vi "Dashboard Main.vi"() -> ()   [LabVIEW 2015]
uses:
  <vilib>/Utility/miscctls.llb/LVRowAndColumnTypeDef.ctl
  <vilib>/event_ctls.llb/eventvkey.ctl
  <vilib>/Rock Robotics/WPI/Dashboard/WPI_DashboardLogging Global.vi
  <vilib>/Rock Robotics/Network Tables/NT Read Numeric Array.vi
  <vilib>/Rock Robotics/Network Tables/NT Read Boolean Array.vi
  <vilib>/Rock Robotics/Network Tables/NT Read Boolean.vi
  <vilib>/Utility/config.llb/Write Key (String).vi
  <vilib>/Utility/config.llb/Write Key (I32).vi
  <vilib>/Utility/config.llb/NI_LVConfig.lvlib
panel:
  in  "TCP":refnum<k5>
  in  "Rec Mode":enum32{"Stop", "Record", "Playback"}(radio)
  in  "Vision":u16(ring)=2 items=["Camera Off", "USB Camera SW", "USB Camera HW", "IP Camera"]
  out "Camera IP":string
  out "Image Message":string="Timeout in Camera Communications"
  in  "Dashboard Tab":T1(tab)
  out "Selected Auto Scheme":string
  out "Gyro":dbl(knob) scale=0.0..360.0
  out "xpos":dbl(slide) scale=-1.0..1.0
  out "target3":bool
  out "target2":bool
  out "target1":bool
  out "NT Connection":bool
  in  "Camera Settings":T2={"Frame Rate"=30, "Compression"=30, "Size"=1} {"Frame Rate" scale=1.0..30.0; "Size" items=["640x480", "320x240", "160x120"]}
  out "MotorChart R":cluster{"Numeric":dbl, "Numeric":dbl}(graph)
  out "MotorChart L":T3(graph)
  out "MotorSliders R":cluster{"MotorSlide1":dbl, "MotorSlide2":dbl} {"MotorSlide2" scale=-1.0..1.0 scale format="%#_2e"; "MotorSlide1" scale=-1.0..1.0 scale format="%#_2e"}
  out "MotorSliders L":T4 {"MotorSlide4 2" scale=0.0..14.0 scale format="%#_2e"; "MotorSlide2" scale=-1.0..1.0 scale format="%#_2e"; "MotorSlide1" scale=-1.0..1.0 scale format="%#_2e"}
  out "JS1 Z":dbl(slide) scale=-1.0..1.0 scale format="%#_2e"
  out "JS1 Graph":cluster{"X":dbl, "Y":dbl}[](graph)
  out "JS1 Buttons":T5
  out "JS2 Z":dbl(slide) scale=-1.0..1.0 scale format="%#_2e"
  out "JS2 Graph":cluster{"X":dbl, "Y":dbl}[](graph)
  out "JS2 Buttons":T5
  out "Mode":T6(ring)=enum."Auto Disabled"
  in  "DB Camera Config":bool
  out "fps":dbl format="%#.1g"
  out "Mbps":dbl format="%#.1g"
  out "Mbps LED":bool
  out "Joystick":bool
  out "Ball":bool
  out "ArmLimit":bool
  out "Intake":bool
  out "Defense":bool
  out "Ldistance":dbl caption="Left"
  out "Rdistance":dbl caption="Right"
  in  "DB/String 9":string
  in  "DB/String 8":string
  in  "DB/String 7":string
  in  "DB/String 6":string
  in  "DB/String 5":string
  in  "DB/String 4":string
  in  "DB/String 3":string
  in  "DB/String 2":string
  in  "DB/String 1":string
  in  "DB/String 0":string
  in  "DB/Slider 0":dbl(slide) scale=0.0..5.0
  in  "DB/Slider 1":dbl(slide) scale=0.0..5.0
  in  "DB/Slider 2":dbl(slide) scale=0.0..5.0
  in  "DB/Slider 3":dbl(slide) scale=0.0..5.0
  out "DB/LED 3":bool
  out "DB/LED 2":bool
  out "DB/LED 1":bool
  out "DB/LED 0":bool
  in  "DB/Button 3":bool
  in  "DB/Button 2":bool
  in  "DB/Button 1":bool
  in  "DB/Button 0":bool caption="New Name"
  in  "BasicAutoParam":dbl[](array[numeric])=[46.0, 95.0, 195.0, 0.5] caption="Auto Params (low bar + others)"
  in  "SelEncoder":bool caption="Use which encoder?"
  in  "Kp":dbl=-0.5 caption="Run straight gain (Kp)"
  in  "Select Auto":string(combo) caption="Select Auto Options"
  in  "idealposition":dbl[](array[numeric])=[8.9, 0.1, 0.08, 0.05] caption="Ideal Position"
  in  "idealspeed":dbl[](array[numeric])=[0.55, 0.55] caption="Ideal Speed"
  out "target":dbl[](array[numeric]) caption="Target"
  in  "Test Slider":dbl(slide) scale=0.0..100.0 scale format="%#_3g"
  in  "On/Off":bool caption="Solenoid"
  in  "Test Name":u16(ring) items=["Select the test to run..."]
  in  "Test Tree":string(tree)
  in  "Motor":cluster{"Value":dbl, "Enable":bool} {"Value" scale=-1.0..1.0 scale format="%#_3g"}
  out "Progress":T7 {"Test Progress" scale=0.0..100.0}
  in  "Rev/Fwd":cluster{"Forward":bool, "Reverse":bool}
  in  "Test Ring":u16(ring) items=["Monochrome", "Color"]
  out "Cmd Status":string
  in  "Execute Command":bool
  in  "Command Params":string[][](table)
  in  "Command Selection":i32(listbox)
  in  "CheckList":i32(listbox)
  out "Tree":string(tree)
  out "Camera Image":T8(plugin-control)
  out "Background":bool
  # "Left"
  # "Front"
  # "Right"
  # "Battery"
  # "Approach distance (auto to defense)"
  # "Breach distance (across defense)"
  # "Travel distance (100\" beyond defense)"
  # "Clockwise turn time (seconds)\nLow bar = 0.5\nRough Terrian / Rock wall = 2.0\nMoat = 3.0"
  # "distance to target"
  # "# targets"
  # "distance to target"
  # "x deadband (close)"
  # "center x"
  # "x center"
  # "center y"
  # "x deadband (far)"
  # "drive speed"
  # "turn speed"
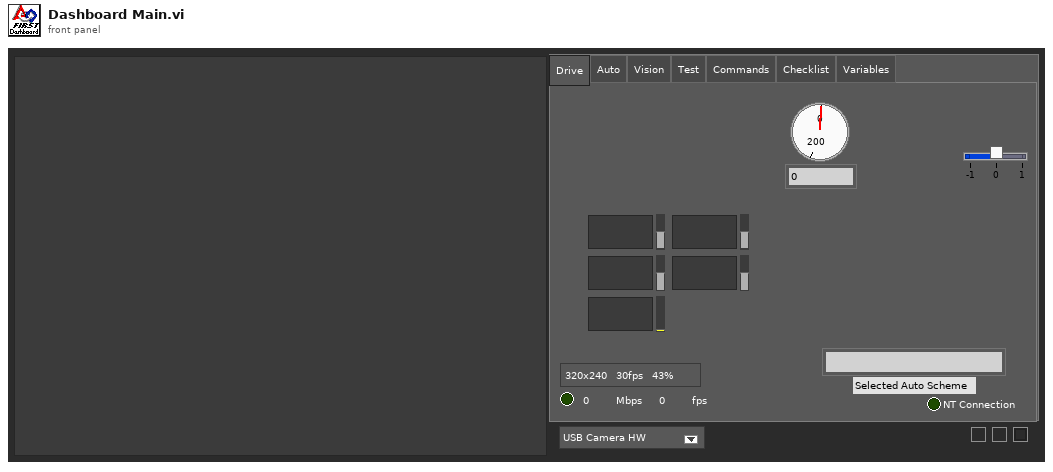
[diagram p1: front panel]
types:
  T1 = enum32{"Drive", "Basic", "Auto", "Vision", "Test", "Commands", "Checklist", "Variables"}
  T2 = cluster{"Frame Rate":i32, "Compression":i32, "Size":u16}
  T3 = cluster{"Numeric":dbl, "Numeric":dbl, "Battery V":dbl}
  T4 = cluster{"MotorSlide1":dbl, "MotorSlide2":dbl, "MotorSlide4 2":dbl}
  T5 = cluster{bool, bool, bool, bool, bool, bool, bool, bool, bool, bool, bool, bool}
  T6 = enum8{"Tele-Op Disabled", "Tele-Op Enabled", "Auto Disabled", "Auto Enabled", "Test Disabled", "Test Enabled", "Disconnected", "No Code", "E-Stop"}
  T7 = cluster{"Test Progress":u8, "Test Progress Text":string}
  T8 = typedef "IMAQ Image.ctl" = refnum<image>
  T9 = cluster{"IDs":cluster{"RPC field ID":u16, "Unique ID":u16}, "String":string}
  T10 = typedef "Image Type" = u32
  T11 = cluster{"Camera Image":refnum<vi>, "Dashboard Tab":refnum<vi>, "Background":refnum<vi>, "Vision":refnum<vi>, "Rec Mode":refnum<vi>, "Test Slider":refnum<vi>, "On/Off ":refnum<vi>, "Test Ring":refnum<vi>, "Rev/Fwd":refnum<vi>, "Test Name":refnum<vi>, "Motor":refnum<vi>, "Progress":refnum<vi>, "CheckList":refnum<vi>, "Tree":refnum<vi>, "Test Tree":refnum<vi>, "Command Params":refnum<vi>, "Command Selection":refnum<vi>, "Execute Command":refnum<vi>, "Cmd Status":refnum<vi>}
  T12 = cluster{"Error Strings":string, "Disable Counts":cluster{u16, u16}, "Rail Faults":cluster{u16, u16, u16}, "Robot IP":string, "DB Mode":u8, "Event Info":cluster{"Name":string, "Type":u8, "Number":u16, "Replay":u8}, "Camera Addr":string}
  T13 = cluster{"Storage":cluster{"Disk Free":u64, "RAM Block":u32, "RAM free":u32}, "CPU Utilization":cluster{"CPU % ISR":sgl, "CPU % Time Crit":sgl, "CPU % Timed Str":sgl, "CPU % High":sgl, "CPU % Above":sgl, "CPU % Normal":sgl, "CPU % Low":sgl}, "CAN":cluster{"% Bus Utilization":sgl, "Bus Off Cnt":u32, "TX_FIFO Full Cnt":u32, "Receive Error Cnt":u8, "Transmit Error Cnt":u8}, "HID":cluster{"HID Outputs":u32, "Rumble Low":u16, "Rumble High":u16}[]}
  T14 = cluster{"Status bits":cluster{"Test Mode":bool, "Autonomous":bool, "Enabled":bool, "Code Start":bool, "Brownout":bool, "Reserved 2":bool, "Reserved 3":bool, "E-Stop":bool}, "Code Trace":cluster{"Disabled":bool, "TeleOp":bool, "Auto":bool, "Test":bool}, "Controller Type":enum16{"unknown", "cRIO", "roboRio"}, "Code?":enum16{"unknown", "noCode", "code"}, "Battery V":dbl}
  T15 = cluster{"Control Bits":cluster{"TestMode":bool, "Autonomous":bool, "Enabled":bool, "FMS Present":bool, bool, bool, bool, "E-Stop":bool}, "Team Station ":u8, "Countdown":sgl, "Joystick Values":cluster{"Axes":dbl[], "Buttons":bool[], "POVs":i16[]}[]}
  T16 = cluster{"Axes":dbl[], "Buttons":bool[], "POVs":i16[]}[]
  T17 = cluster{"Axes":dbl[], "Buttons":bool[], "POVs":i16[]}
  T18 = cluster{"Buttons[0]":bool, "Buttons[1]":bool, "Buttons[2]":bool, "Buttons[3]":bool, "Buttons[4]":bool, "Buttons[5]":bool, "Buttons[6]":bool, "Buttons[7]":bool, "Buttons[8]":bool, "Buttons[9]":bool, "Buttons[10]":bool, "Buttons[11]":bool}
  T19 = typedef "NI_LVConfig.lvlib/Config Data RefNum.ctl" = refnum<k1>
  T20 = cluster{"Operation":enum16{"Update", "Clear"}, "Color Box":u32}[]
  T21 = typedef "eventvkey.ctl" = enum16{"ASCII", "Enter", "Return", "Shift", "Ctrl", "Alt", "Cmd", "Opt", "Caps", "NumLock", "Clear", "Break", "Up", "Down", "Left", "Right", "Insert", "Delete", "Home", "End", "PageUp", "PageDown", "Escape", "Help", "Pause", "ScrollLock", "F1", "F2", "F3", "F4", "F5", "F6", "F7", "F8", "F9", "F10", "F11", "F12", "F13", "F14", "F15", "F16", "F17", "F18", "F19", "F20", "F21", "F22", "F23", "F24", "Play", "VolumeUp", "VolumeDown", "Mute", "Two Byte Char"}
  T22 = cluster{"Image Size":bool, "Image Type":bool, "Pixel Value":bool, "ROI Information":bool, "Zoom Factor":bool}
  T23 = enum8{"Enabled", "Disabled", "Disabled and Grayed Out"}
  T24 = cluster{"Operation":enum16{"Update", "Clear"}, "Color Box":u32}
  T25 = typedef "LVRowAndColumnTypeDef.ctl" = cluster{"Row":i32, "Column":i32}
  T26 = cluster{"Shift":bool, "Ctrl":bool, "Alt":bool, "Cmd":bool, "Opt":bool}
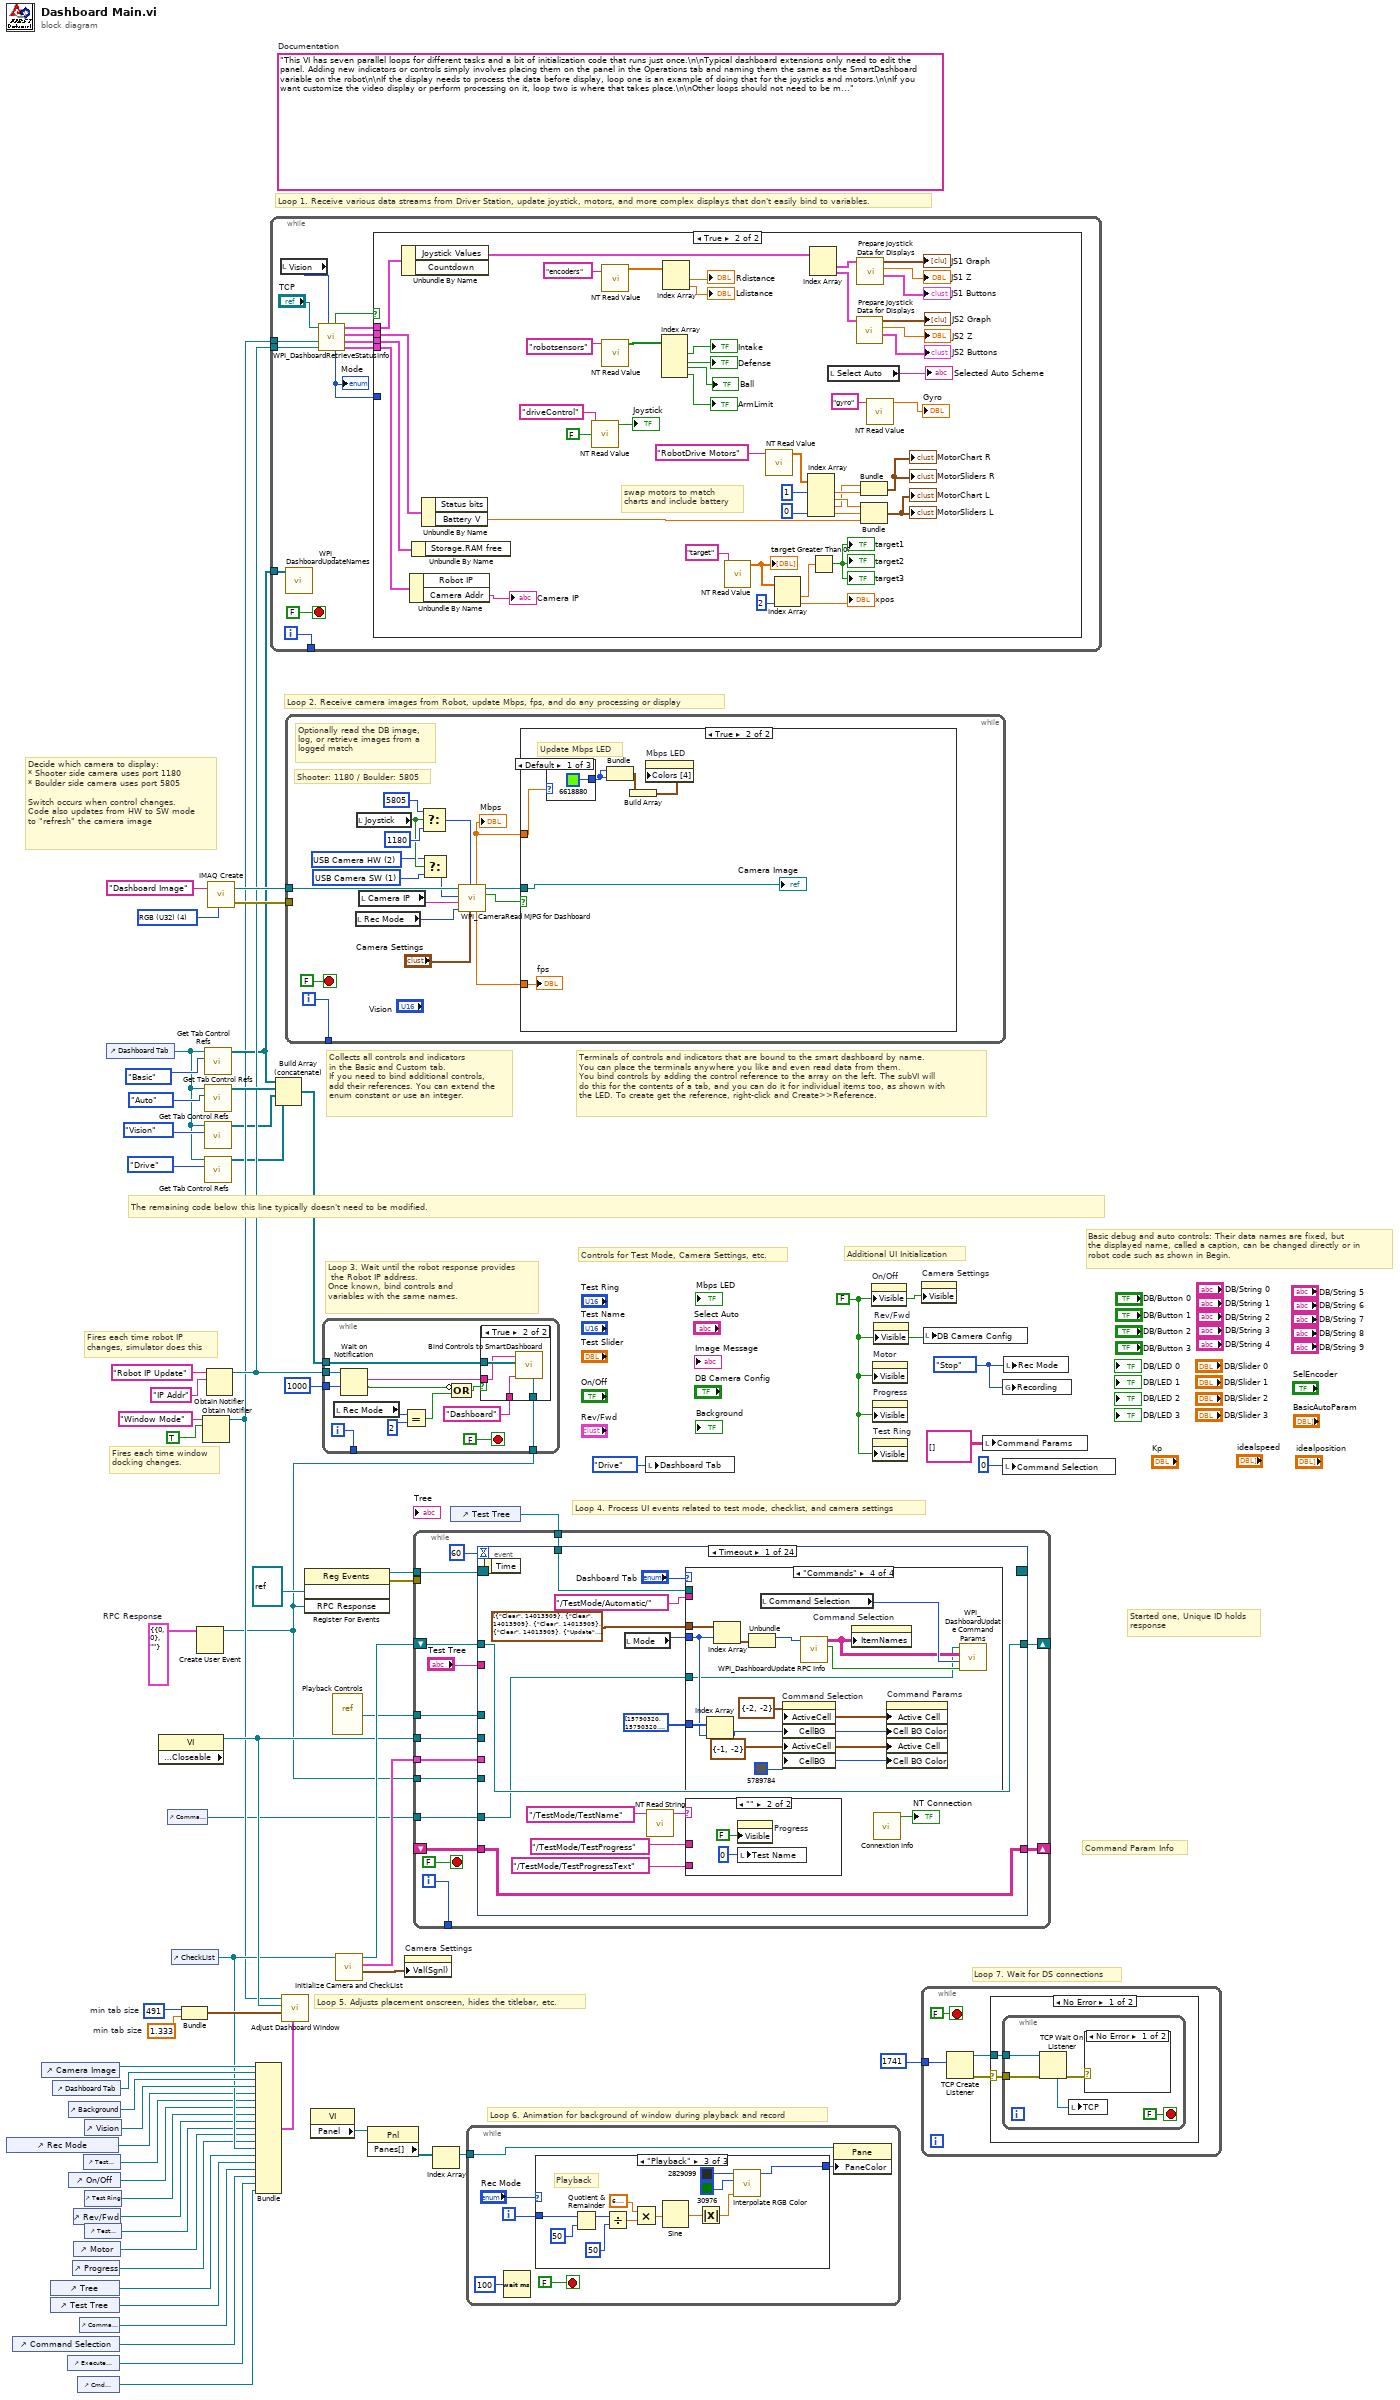
[diagram p0: block diagram]
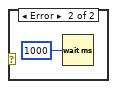
[diagram p2: hidden frame]
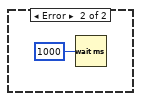
[diagram p3: hidden frame]
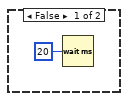
[diagram p4: hidden frame]
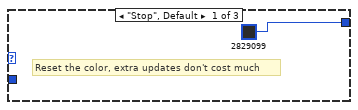
[diagram p5: hidden frame]
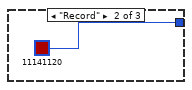
[diagram p6: hidden frame]
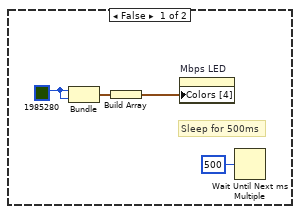
[diagram p8: hidden frame]
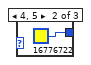
[diagram p9: hidden frame]
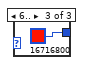
[diagram p10: hidden frame]
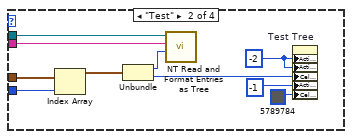
[diagram p12: hidden frame]
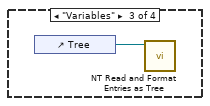
[diagram p13: hidden frame]
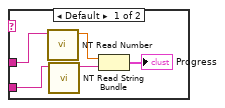
[diagram p14: hidden frame]
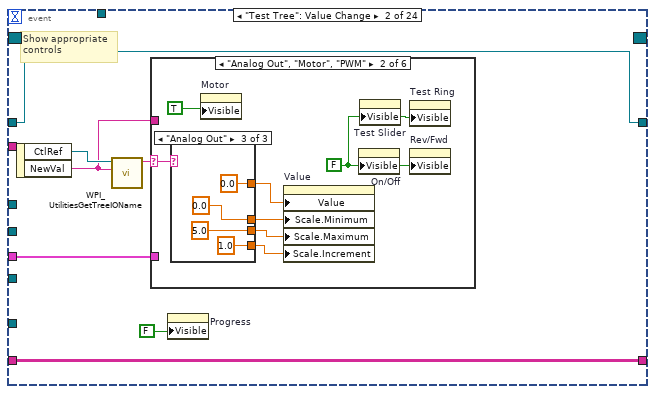
[diagram p15: hidden frame]
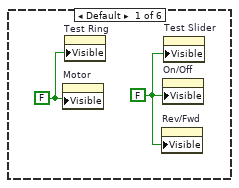
[diagram p16: hidden frame]
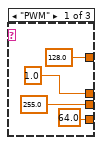
[diagram p17: hidden frame]
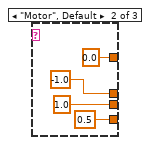
[diagram p18: hidden frame]
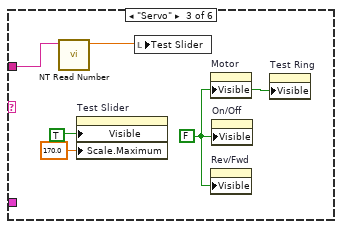
[diagram p19: hidden frame]
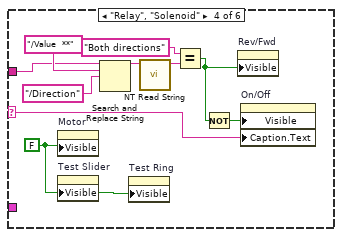
[diagram p20: hidden frame]
diagram:
  w15 = T9 {"IDs"={"RPC field ID"=0, "Unique ID"=0}, "String"=""}  # RPC Response
  w38 = 491  # min tab size
  w37 = 1.333  # min tab size
  w45 = enum32{"Stop", "Record", "Playback"}."Stop" ("Rec Mode")
  w22 = FALSE ("Visible")
  (unwired) "This VI has seven parallel loops for different tasks and a bit of initialization code that runs just once.\n\nTypical dashboard extensions only need to edit the panel. Adding new indicators or controls simply involves placing them on the panel in the Operations tab and naming them the same as the SmartDashboard variable on the robot\n\nIf the display needs to process the data before display, loop one is an example of doing that for the joysticks and motors.\n\nIf you want customize the video display or perform processing on it, loop two is where that takes place.\n\nOther loops should not need to be modified. They are pretty standard, and document the task they perform."  # Documentation
  w65 = T10 4 items=["Grayscale (U8)", "Grayscale (I16)", "Grayscale (SGL)", "Complex (CSG)", "RGB (U32)", "HSL (U32)", "RGB (U64)"] ("Image Type")
  # "Decide which camera to display:\n* Shooter side camera uses port 1180\n* Boulder side camera uses port 5805\n\nSwitch occurs when control changes.\nCode also updates from HW to SW mode\nto \"refresh\" the camera image"
  # "Command Param Info"
  # "Started one, Unique ID holds\nresponse"
  # "Loop 7. Wait for DS connections"
  # "Basic debug and auto controls: Their data names are fixed, but\nthe displayed name, called a caption, can be changed directly or in\nrobot code such as shown in Begin."
  # "Controls for Test Mode, Camera Settings, etc."
  # "Additional UI Initialization"
  # "Loop 6. Animation for background of window during playback and record"
  # "Fires each time robot IP\nchanges, simulator does this"
  # "Fires each time window\ndocking changes."
  # "Collects all controls and indicators\nin the Basic and Custom tab.\nIf you need to bind additional controls,\nadd their references. You can extend the\nenum constant or use an integer."
  # "The remaining code below this line typically doesn't need to be modified."
  # "Loop 4. Process UI events related to test mode, checklist, and camera settings"
  # "Terminals of controls and indicators that are bound to the smart dashboard by name.\nYou can place the terminals anywhere you like and even read data from them.\nYou bind controls by adding the control reference to the array on the left. The subVI will\ndo this for the contents of a tab, and you can do it for individual items too, as shown with\nthe LED. To create get the reference, right-click and Create>>Reference."
  # "Loop 3. Wait until the robot response provides\n the Robot IP address.\nOnce known, bind controls and\nvariables with the same names."
  # "Loop 5. Adjusts placement onscreen, hides the titlebar, etc."
  # "Loop 1. Receive various data streams from Driver Station, update joystick, motors, and more complex displays that don't easily bind to variables."
  # "Loop 2. Receive camera images from Robot, update Mbps, fps, and do any processing or display"
  n1 = control-ref of="Rec Mode"() -> (w28:refnum<vi>)
  n2 = control-ref of="Command Selection"() -> (w14:refnum<vi>)
  n3 = control-ref of="Camera Image"() -> (w41:refnum<vi>)
  n4 = control-ref of="Tree"() -> (w32:refnum<vi>)
  n5 = control-ref of="Test Tree"() -> (w31:refnum<vi>)
  n6 = control-ref of="Dashboard Tab"() -> (w40:refnum<vi>)
  n7 = control-ref of="Execute Command"() -> (w16:refnum<vi>)
  n8 = control-ref of="Background"() -> (w35:refnum<vi>)
  n9 = control-ref of="On/Off"() -> (w26:refnum<vi>)
  n10 = control-ref of="Progress"() -> (w23:refnum<vi>)
  n11 = control-ref of="Rev/Fwd"() -> (w24:refnum<vi>)
  n12 = control-ref of="Motor"() -> (w29:refnum<vi>)
  n13 = control-ref of="Cmd Status"() -> (w10:refnum<vi>)
  n14 = control-ref of="Command Params"() -> (w17:refnum<vi>)
  n15 = control-ref of="Test Slider"() -> (w27:refnum<vi>)
  n16 = control-ref of="Vision"() -> (w39:refnum<vi>)
  n17 = control-ref of="Test Ring"() -> (w25:refnum<vi>)
  n18 = control-ref of="Test Name"() -> (w30:refnum<vi>)
  n19 = control-ref of="Dashboard Tab"() -> (w2:refnum<vi>)
  n20 = property class="VI" props=["Front Panel.Closeable"]() -> (reference out=w44:refnum<vi>)  [unwired: 2 in, 2 out]
  n21 = control-ref of="Command Params"() -> (w9:refnum<vi>)
  n22 = control-ref of="CheckList"() -> (w33:refnum<vi>)
  n23 = Bundle("min tab size"=w38, "min tab size"=w37) -> (w36:cluster{"min tab size":i32, "min tab size":dbl})  [unwired: 1 in]
  n24 = Create User Event(user event datatype=w15) -> (user event=w11:refnum<user-event>)  [unwired: 1 in, 1 out]
  n25 = Obtain Notifier(name (unnamed)="Window Mode", notification data type=TRUE) -> (notifier out=w19:refnum<notifier>)  [unwired: 2 in, 2 out]
  n26 = call <vilib>:"Get Tab Control Refs.vi"("Page Index"=T1."Basic" ("Dashboard Tab"), "TabControl in"=w2) -> ("ControlsOnPage"=w20:refnum<vi>[])  [unwired: 9 in]
  n27 = call <vilib>:"Get Tab Control Refs.vi"("Page Index"=T1."Auto" ("Dashboard Tab"), "TabControl in"=w2) -> ("ControlsOnPage"=w43:refnum<vi>[])  [unwired: 9 in]
  n28 = call <vilib>:"Get Tab Control Refs.vi"("Page Index"=T1."Vision" ("Dashboard Tab"), "TabControl in"=w2) -> ("ControlsOnPage"=w4:refnum<vi>[])  [unwired: 9 in]
  n29 = call <vilib>:"Get Tab Control Refs.vi"("Page Index"=T1."Drive" ("Dashboard Tab"), "TabControl in"=w2) -> ("ControlsOnPage"=w1:refnum<vi>[])  [unwired: 9 in]
  n30 = Obtain Notifier(name (unnamed)="Robot IP Update", notification data type="IP Addr" ("name (unnamed)")) -> (notifier out=w21:refnum<notifier>)  [unwired: 2 in, 2 out]
  n31 = call "IMAQ Create"("Image Name"="Dashboard Image", "Image Type"=w65) -> ("New Image"=w63:T8, "error out"=w62:errorcluster)  [unwired: 2 in, 1 out]
  n32 = Bundle("Camera Image"=w41, "Dashboard Tab"=w40, "Background"=w35, "Vision"=w39, "Rec Mode"=w28, "Test Slider"=w27, "On/Off"=w26, "Test Ring"=w25, "Rev/Fwd"=w24, "Test Name"=w30, "Motor"=w29, "Progress"=w23, "CheckList"=w33, "Tree"=w32, "Test Tree"=w31, "Command Params"=w17, "Command Selection"=w14, "Execute Command"=w16, "Cmd Status"=w10) -> (w34:T11)  [unwired: 1 in]
  n33 = while {
    tunnel: [w77] -> _
    tunnel: w21 -> [w71]
    tunnel: w20 -> [w70]
    tunnel: w19 -> [w66]
    i -> [w77]
    stop <- FALSE stop-if-true
    n34 = local read "Vision"() -> (w68:u16)
    n35 = call <vilib>:"WPI_DashboardUpdateNames.vi"("Controls on Tab"=w70) -> ()  [unwired: 11 in]
    n36 = call <vilib>:"WPI_DashboardRetrieveStatusInfo.vi"("Vision"=w68, "Binding Refnum"=w71, "Window Mode Notifier"=w66, "TCP Cnx"="TCP") -> ("Power and Errors"=w72:T12, "Robot Metrics"=w75:T13, "Status Info"=w76:T14, "Control Info"=w73:T15, "Robot Mode"=w69:T6, "Process?"=w74:bool)  [unwired: 2 in]
    "Mode" <- w69
    n37 = case shown="True" w74 {
      tunnel: w76 -> [_ w126]
      tunnel: w75 -> [_ w125]
      tunnel: w73 -> [_ w124]
      tunnel: w72 -> [_ w123]
      tunnel: w69 -> [_ _]
      frame False {
        n38 = Wait (ms)(milliseconds to wait=u32 20) -> ()  [unwired: 1 out]
      }
      frame True {
        # "swap motors to match\ncharts and include battery"
        n39 = Unbundle By Name(w124) -> ("Joystick Values"=w113:T16)  [unwired: 1 out]
        n40 = Unbundle By Name(w123) -> ("Camera Addr"=→"Camera IP":string)  [unwired: 1 out]
        n41 = Unbundle By Name(w125) -> ()  [unwired: 1 out]
        n42 = Unbundle By Name(w126) -> ("Battery V"=w114:dbl)  [unwired: 1 out]
        n43 = call-poly <vilib>:"NT Read Value.vi"("Default Value"=FALSE, "Name"="driveControl") -> ("Boolean"=→"Joystick":bool)  [unwired: 8 in, 1 out]
        n44 = call-poly <vilib>:"NT Read Value.vi"("Name"="encoders") -> ("Numeric Array"=w100:dbl[])  [unwired: 9 in, 1 out]
        n45 = call-poly <vilib>:"NT Read Value.vi"("Name"="robotsensors") -> ("Boolean Array"=w98:bool[])  [unwired: 9 in, 1 out]
        n46 = Index Array(array=w98) -> (element #1=→"Intake":bool, element #2=→"Defense":bool, element #3=→"Ball":bool, element #4=→"ArmLimit":bool)  [unwired: 4 in]
        n47 = Index Array(array=w100) -> (element #1=→"Rdistance":dbl, element #2=→"Ldistance":dbl)  [unwired: 2 in]
        n48 = call-poly <vilib>:"NT Read Value.vi"("Name"="target") -> ("Numeric Array"=w87:dbl[])  [unwired: 9 in, 1 out]
        "target" <- w87
        n49 = call-poly <vilib>:"NT Read Value.vi"("Name"="RobotDrive Motors") -> ("Numeric Array"=w102:dbl[])  [unwired: 9 in, 1 out]
        n50 = Index Array(array=w87, index #2=2 ("index")) -> (element #1=w86:dbl, element #2=→"xpos":dbl)  [unwired: 1 in]
        n51 = Index Array(array=w102, index #1=1, index #4=0) -> (element #1=w118:dbl, element #2=w119:dbl, element #3=w117:dbl, element #4=w122:dbl)  [unwired: 2 in]
        n52 = Index Array(array=w113) -> (element #1=w112:T17, element #2=w107:T17)  [unwired: 2 in]
        n53 = Greater Than 0?(x=w86) -> (x > 0?=→"target1" →"target2" →"target3":bool)
        n54 = local read "Select Auto"() -> (→"Selected Auto Scheme":string)
        n55 = call "Prepare Joystick Data for Displays.vi"("Joystick Values"=w107) -> ("Buttons"=→"JS2 Buttons":T18, "Z Axis"=→"JS2 Z":dbl, "Cartesian Data"=→"JS2 Graph":cluster{"X axis":dbl, "X axis":dbl}[])  [unwired: 8 in]
        n56 = call "Prepare Joystick Data for Displays.vi"("Joystick Values"=w112) -> ("Buttons"=→"JS1 Buttons":T18, "Z Axis"=→"JS1 Z":dbl, "Cartesian Data"=→"JS1 Graph":cluster{"X axis":dbl, "X axis":dbl}[])  [unwired: 8 in]
        n57 = Bundle("Numeric"=w117, "Numeric"=w118) -> (→"MotorChart R" →"MotorSliders R":cluster{"Numeric":dbl, "Numeric":dbl})  [unwired: 1 in]
        n58 = Bundle("Numeric"=w119, "Numeric"=w122, "Battery V"=w114) -> (→"MotorChart L" →"MotorSliders L":T3)  [unwired: 1 in]
        n59 = call-poly <vilib>:"NT Read Value.vi"("Name"="gyro") -> ("Numeric"=→"Gyro":dbl)  [unwired: 9 in, 1 out]
      }
    }
  }
  n60 = Build Array (concatenate)(w20, w43, w4, w1) -> (w42:refnum<vi>[])
  n61 = call "Adjust Dashboard Window.vi"("Sizing Refnums"=w34, "Size Constraints"=w36, "VI"=w44, "WIn Mode"=w19) -> ()  [unwired: 8 in]
  n62 = while {
    tunnel: w63 -> [w141]
    tunnel: w62 -> [_]
    tunnel: [w142] -> _
    i -> [w142]
    stop <- FALSE stop-if-true
    w128 = u16 1 items=["Camera Off", "USB Camera SW", "USB Camera HW", "IP Camera"] ("Vision 2")
    w127 = u16 2 items=["Camera Off", "USB Camera SW", "USB Camera HW", "IP Camera"] ("Vision 2")
    # "Shooter: 1180 / Boulder: 5805"
    # "Optionally read the DB image,\nlog, or retrieve images from a\nlogged match"
    n63 = local read "Rec Mode"() -> (w136:enum32{"Stop", "Record", "Playback"})
    n64 = local read "Joystick"() -> (w130:bool)
    n65 = local read "Camera IP"() -> (w135:string)
    n66 = Select(t=u16 5805 ("port"), s=w130, f=u16 1180 ("port")) -> (s? t:f=w131:u16)
    n67 = Select(t=w127, s=w130, f=w128) -> (s? t:f=w129:u16)
    n68 = call "WPI_CameraRead MJPG for Dashboard.vi"("Camera Settings"="Camera Settings", "port"=w131, "Rec Mode"=w136, "Camera IP"=w135, "Camera Mode"=w129, "Refnum in"=w141) -> ("Active"=w139:bool, "Refnum out"=w140:T8, "FPS"=w138:dbl, "Bandwidth (Mbps)"=w134:dbl)  [unwired: 2 in]
    "Mbps" <- w134
    n69 = case shown="True" w139 {
      tunnel: w140 -> [_ w148]
      tunnel: w134 -> [_ w150]
      tunnel: w138 -> [_ w149]
      frame False {
        w144 = u32 1985280 ("Color Box")
        # "Sleep for 500ms"
        n70 = Bundle("Color Box"=w144, "Color Box"=w144) -> (w146:cluster{"Color Box":u32, "Color Box":u32})  [unwired: 1 out]
        n71 = Build Array(w146) -> (w145:cluster{"Color Box":u32, "Color Box":u32}[])
        n72 = property on="Mbps LED" class="Bool (strict)"("Colors [4]"=w145) -> ()  [unwired: 2 in, 2 out]
        n73 = Wait Until Next ms Multiple(millisecond multiple=u32 500) -> ()  [unwired: 1 out]
      }
      frame True {
        # "Update Mbps LED"
        n74 = case shown="Default" w150 {
          tunnel: [u32 6618880 ("Color Box") u32 16776722 ("Color Box") u32 16716800 ("Color Box")] -> w151
          frame Default {
          }
          frame 4, 5 {
          }
          frame 6.. {
          }
        }
        n75 = Bundle("Color Box"=w151, "Color Box"=w151) -> (w153:cluster{"Color Box":u32, "Color Box":u32})  [unwired: 1 out]
        n76 = Build Array(w153) -> (w152:cluster{"Color Box":u32, "Color Box":u32}[])
        n77 = property on="Mbps LED" class="Bool (strict)"("Colors [4]"=w152) -> ()  [unwired: 2 in, 2 out]
        "fps" <- w149
        "Camera Image" <- w148
      }
    }
  }
  n78 = register-events(refnum<vi> refnum, w11) -> (reference out=w49:refnum<event-registration>, error out=w48:errorcluster)  [unwired: 2 in]
  n79 = property class="VI"() -> ("Panel"=w52:refnum<vi>)  [unwired: 2 in, 2 out]
  n80 = while {
    tunnel: w42 -> [w169]
    tunnel: w21 -> [w167]
    tunnel: [w165] -> _
    tunnel: u32 1000 ("milliseconds to wait") -> [w164]
    tunnel: w11 -> [w157]
    i -> [w165]
    stop <- FALSE stop-if-true
    n81 = local read "Rec Mode"() -> (w160:enum32{"Stop", "Record", "Playback"})
    n82 = Wait on Notification(notifier=w167, timeout in ms (-1)=w164) -> (notification=w166:string, timed out?=w162:bool)  [unwired: 2 in, 2 out]
    n83 = Equal?(x=w160, y=u16 2 ("Rec Mode")) -> (x = y?=w161:bool)
    n84 = Compound Arithmetic op=OR(invert w162, w161) -> (w163:bool)
    n85 = case shown="True" w163 {
      tunnel: w169 -> [_ w173]
      tunnel: w166 -> [_ w172]
      tunnel: "Dashboard" -> [_ w171]
      tunnel: w157 -> [_ w170]
      frame False {
      }
      frame True {
        n86 = call <vilib>:"Bind Controls to SmartDashboard.vi"("RPC ref"=w170, "Client Name"=w171, "Bound Control Refs"=w173, "Server IP Address"=w172) -> ()  [unwired: 8 in]
      }
    }
  }
  n87 = vi-ref "Playback Controls.vi"() -> (w50:refnum<vi>)
  n88 = call "Initialize Camera and CheckList.vi"("ListBox in"=w33) -> ("Cluster"=w56:cluster{"value":i32, "value":i32, "index":i32}, "Array"=w57:cluster{string[]}[], "File Refnum"=w55:T19)  [unwired: 8 in]
  n89 = property class="Pnl"(reference=w52) -> ("Panes[]"=w53:refnum<vi>[])  [unwired: 1 in, 2 out]
  n90 = property on="Camera Settings" class="Clust (strict)"("Val(Sgnl)"=w56) -> ()  [unwired: 2 in, 2 out]
  n91 = Index Array(array=w53) -> (element=w51:refnum<vi>)  [unwired: 1 in]
  n92 = control-ref of="Test Tree"() -> (w54:refnum<vi>)
  n93 = while {
    tunnel: w57 -> [w185]
    shift-right: [w184] -> _
    shift-left: w55 -> [w183]
    tunnel: [w182] -> _
    tunnel: w54 -> [w181]
    tunnel: w50 -> [w180]
    tunnel: w49 -> [w179]
    tunnel: w48 -> [_]
    tunnel: w44 -> [w178]
    tunnel: w11 -> [w177]
    tunnel: w9 -> [w176]
    shift-right: [w175] -> _
    shift-left: _ -> [w174]
    i -> [w182]
    stop <- FALSE stop-if-true
    n94 = event shown="[0] Timeout" {
      selector: w179 -> [_ _ _ _ _ _ _ _ _ _ _ _ _ _ _ _ _ _ _ _ _ _ _ _]
      dyn-events: [_ _ _ _ _ _ _ _ _ _ _ _ _ _ _ _ _ _ w494 _ _ _ _ _] -> _
      timeout: u32 60 ("milliseconds to wait") -> [_ _ _ _ _ _ _ _ _ _ _ _ _ _ _ _ _ _ _ _ _ _ _ _]
      tunnel: w181 -> [w198 _ _ _ _ _ _ _ _ _ _ _ _ _ _ _ _ _ _ _ _ _ _ _]
      tunnel: "Test Tree" -> [_ _ _ _ _ _ _ _ _ _ _ _ _ w457 w466 w469 w474 w483 _ _ _ _ _ _]
      tunnel: w185 -> [_ w236 _ _ _ _ _ _ _ _ _ w419 w450 _ _ _ _ _ _ _ _ _ _ _]
      tunnel: [w195 w235 w339 w345 w355 w359 w365 w377 w385 w391 w404 w418 w443 w456 w464 w468 w473 w482 w496 w512 w514 w522 w533 w538] -> w184
      tunnel: w183 -> [w195 w235 w339 w345 w355 w359 w365 w377 w385 w391 w404 w417 w443 w456 w464 w468 w473 w482 w496 w512 w514 w522 w533 w538]
      tunnel: w180 -> [_ _ _ _ _ _ _ _ _ _ _ _ _ _ _ _ _ _ w497 _ w517 _ _ _]
      tunnel: w178 -> [_ _ _ _ _ _ _ _ _ _ _ _ _ _ _ _ _ _ w492 _ _ _ _ _]
      tunnel: w177 -> [_ _ _ _ _ _ _ _ _ _ _ _ _ _ _ _ _ _ w488 _ _ _ _ _]
      tunnel: w176 -> [w190 _ _ _ _ _ w363 _ _ _ _ _ _ _ _ _ _ _ _ _ _ _ _ _]
      tunnel: [w189 w234 w338 w344 w354 w360 w361 w371 w382 w390 w403 w416 w442 w455 w463 w467 w472 w481 w487 w510 w513 w518 w526 w539] -> w175
      tunnel: w174 -> [w189 w234 w338 w344 w354 w360 w361 _ _ w390 w403 w416 w442 w455 w463 w467 w472 w481 w487 w510 w513 w518 w526 w539]
      event Timeout {
        n95 = event-data() -> ()  [unwired: 1 in, 1 out]
        n96 = local read "Mode"() -> (w192:T6)
        n97 = call <vilib>:"NT Read String.vi"("Name"="/TestMode/TestName") -> ("String"=w201:string)  [unwired: 9 in, 1 out]
        n98 = case shown="\"Commands\"" "Dashboard Tab" {
          tunnel: w198 -> [_ w212 _ _]
          tunnel: "/TestMode/Automatic/" ("Name Pattern") -> [_ w211 _ _]
          tunnel: T20 [{"Operation"=enum."Clear", "Color Box"=14013909}, {"Operation"=enum."Clear", "Color Box"=14013909}, {"Operation"=enum."Clear", "Color Box"=14013909}, {"Operation"=enum."Clear", "Color Box"=14013909}, {"Operation"=enum."Update", "Color Box"=14013909}, {"Operation"=enum."Update", "Color Box"=16777215}, {"Operation"=enum."Clear", "Color Box"=14013909}, {"Operation"=enum."Clear", "Color Box"=14013909}, {"Operation"=enum."Clear", "Color Box"=14013909}] -> [_ w204 _ w221]
          tunnel: w192 -> [_ w203 _ w220]
          tunnel: u32[] [15790320, 15790320, 15790320, 15790320, 16777215, 16777215, 15790320, 15790320, 15790320] -> [_ _ _ w226]
          tunnel: w190 -> [_ _ _ w214]
          frame "Auto", Default {
          }
          frame "Test" {
            w210 = -2 ("Active Item:Row Number")
            n99 = Index Array(array=w204, index=w203) -> (element=w205:T24)
            n100 = Unbundle(w205) -> ("Operation"=w206:enum16{"Update", "Clear"}, "Color Box"=w207:u32)
            n101 = call <vilib>:"NT Read and Format Entries as Tree.vi"("Operation"=w206, "Name Pattern"=w211, "Tree Refnum"=w212) -> ()  [unwired: 7 in, 2 out]
            n102 = property on="Test Tree" class="Tree (strict)"("Active Item Row Number"=w210, "ActiveColNum"=w210, "CellBG"=w207, "Active Item Row Number"=-1 ("Active Item:Row Number"), "CellBG"=u32 5789784 ("Color Box")) -> ()  [unwired: 2 in, 2 out]
          }
          frame "Variables" {
            n103 = control-ref of="Tree"() -> (w213:refnum<vi>)
            n104 = call <vilib>:"NT Read and Format Entries as Tree.vi"("Tree Refnum"=w213) -> ()  [unwired: 9 in, 2 out]
          }
          frame "Commands" {
            w222 = u32 5789784 ("Color Box")
            w223 = T25 {"Row"=-1, "Column"=-2} ("Active Cell:Active Cell")
            w225 = T25 {"Row"=-2, "Column"=-2} ("Active Cell:Active Cell")
            n105 = Index Array(array=w226, index=w220) -> (element=w224:u32)
            n106 = Index Array(array=w221, index=w220) -> (element=w219:T24)
            n107 = Unbundle(w219) -> ("Operation"=w218:enum16{"Update", "Clear"})  [unwired: 1 out]
            n108 = local read "Command Selection"() -> (w217:i32)
            n109 = property on="Command Selection" class="MCListbox (strict)"("ActiveCell"=w225, "CellBG"=w224, "ActiveCell"=w223, "CellBG"=w222) -> ()  [unwired: 2 in, 2 out]
            n110 = call <vilib>:"WPI_DashboardUpdate RPC Info.vi"("Operation"=w218) -> ("update"=w216:bool, "commands"=w215:string[][])  [unwired: 9 in]
            n111 = property on="Command Selection" class="MCListbox (strict)"("ItemNames"=w215) -> ()  [unwired: 2 in, 2 out]
            n112 = property on="Command Params" class="Tbl (strict)"("Active Cell"=w225, "Cell BG Color"=w224, "Active Cell"=w223, "Cell BG Color"=w222) -> ()  [unwired: 2 in, 2 out]
            n113 = call <vilib>:"WPI_DashboardUpdate Command Params.vi"("Update"=w216, "NewVal"=w217, "Commands"=w215, "Param Tbl"=w214) -> ()  [unwired: 7 in, 1 out]
          }
        }
        n114 = case shown="\"\"" w201 {
          tunnel: "/TestMode/TestProgress" ("Name") -> [w228 _]
          tunnel: "/TestMode/TestProgressText" ("Name") -> [w227 _]
          frame Default {
            n115 = call <vilib>:"NT Read Number.vi"("Name"=w228) -> ("Numeric"=w229:dbl)  [unwired: 9 in, 1 out]
            n116 = call <vilib>:"NT Read String.vi"("Name"=w227) -> ("String"=w230:string)  [unwired: 9 in, 1 out]
            n117 = Bundle("Numeric"=w229, "String"=w230) -> (→"Progress":cluster{"Numeric":dbl, "String":string})  [unwired: 1 in]
          }
          frame "" {
            n118 = property on="Progress" class="Clust (strict)"("Visible"=FALSE) -> ()  [unwired: 2 in, 2 out]
            n119 = local write "Test Name"(u16 0) -> ()
          }
        }
        n120 = call <vilib>:"Connextion Info.vi"() -> ("Connected"=→"NT Connection":bool)  [unwired: 10 in, 1 out]
      }
      event "Test Tree": Value Change {
        # "Show appropriate\ncontrols"
        n121 = event-data() -> ("CtlRef"=w239:refnum<vi>, "NewVal"=w237:string)  [unwired: 1 in]
        n122 = call <vilib>:"WPI_UtilitiesGetTreeIOName.vi"("NewVal"=w237, "TreeControl in"=w239) -> ("I/O Name"=w240:string)  [unwired: 9 in]
        n123 = case shown="\"Analog Out\", \"Motor\", \"PWM\"" w240 {
          selector: w240 -> [_ w247 _ w269 w278 _]
          tunnel: w237 -> [_ _ w266 w268 _ w285]
          tunnel: w236 -> [_ _ _ _ _ w284]
          frame Default {
            w242 = FALSE ("Visible")
            w241 = FALSE ("Visible")
            n124 = property on="Motor" class="Clust (strict)"("Visible"=w241) -> ()  [unwired: 2 in, 2 out]
            n125 = property on="Test Ring" class="Ring (strict)"("Visible"=w241) -> ()  [unwired: 2 in, 2 out]
            n126 = property on="Rev/Fwd" class="Clust (strict)"("Visible"=w242) -> ()  [unwired: 2 in, 2 out]
            n127 = property on="On/Off" class="Bool (strict)"("Visible"=w242) -> ()  [unwired: 2 in, 2 out]
            n128 = property on="Test Slider" class="Slide (strict)"("Visible"=w242) -> ()  [unwired: 2 in, 2 out]
          }
          frame "Analog Out", "Motor", "PWM" {
            w248 = FALSE ("Visible")
            n129 = case shown="\"Analog Out\"" w247 {
              tunnel: [1.0 ("Value") -1.0 ("Value") 0.0 ("Value")] -> w246
              tunnel: [255.0 ("Value") 1.0 ("Value") 5.0 ("Value")] -> w245
              tunnel: [128.0 ("Value") 0.0 ("Value") 0.0 ("Value")] -> w244
              tunnel: [64.0 ("Value") 0.5 ("Value") 1.0 ("Value")] -> w243
              frame "PWM" {
              }
              frame "Motor", Default {
              }
              frame "Analog Out" {
              }
            }
            n130 = property on="Motor" class="Clust (strict)"("Visible"=TRUE) -> ()  [unwired: 2 in, 2 out]
            n131 = property on="Value" class="Slide (strict)"("Value"=w244, "Scale.Minimum"=w246, "Scale.Maximum"=w245, "Scale.Increment"=w243) -> ()  [unwired: 2 in, 2 out]
            n132 = property on="On/Off" class="Bool (strict)"("Visible"=w248) -> ()  [unwired: 2 in, 2 out]
            n133 = property on="Test Slider" class="Slide (strict)"("Visible"=w248) -> ()  [unwired: 2 in, 2 out]
            n134 = property on="Test Ring" class="Ring (strict)"("Visible"=w248) -> ()  [unwired: 2 in, 2 out]
            n135 = property on="Rev/Fwd" class="Clust (strict)"("Visible"=w248) -> ()  [unwired: 2 in, 2 out]
          }
          frame "Servo" {
            w264 = FALSE ("Visible")
            n136 = call <vilib>:"NT Read Number.vi"("Name"=w266) -> ("Numeric"=w265:dbl)  [unwired: 9 in, 1 out]
            n137 = property on="Test Slider" class="Slide (strict)"("Visible"=TRUE, "Scale.Maximum"=170.0 ("Scale.Range:Maximum")) -> ()  [unwired: 2 in, 2 out]
            n138 = local write "Test Slider"(w265) -> ()
            n139 = property on="Motor" class="Clust (strict)"("Visible"=w264) -> ()  [unwired: 2 in, 2 out]
            n140 = property on="Rev/Fwd" class="Clust (strict)"("Visible"=w264) -> ()  [unwired: 2 in, 2 out]
            n141 = property on="On/Off" class="Bool (strict)"("Visible"=w264) -> ()  [unwired: 2 in, 2 out]
            n142 = property on="Test Ring" class="Ring (strict)"("Visible"=w264) -> ()  [unwired: 2 in, 2 out]
          }
          frame "Relay", "Solenoid" {
            w267 = FALSE ("Visible")
            n143 = property on="Motor" class="Clust (strict)"("Visible"=w267) -> ()  [unwired: 2 in, 2 out]
            n144 = property on="Test Slider" class="Slide (strict)"("Visible"=w267) -> ()  [unwired: 2 in, 2 out]
            n145 = Search and Replace String(input string=w268, search string="/Value  **", replace string="/Direction") -> (result string=w274:string)  [unwired: 5 in, 3 out]
            n146 = property on="Test Ring" class="Ring (strict)"("Visible"=w267) -> ()  [unwired: 2 in, 2 out]
            n147 = call <vilib>:"NT Read String.vi"("Name"=w274) -> ("String"=w272:string)  [unwired: 9 in, 1 out]
            n148 = Equal?(x="Both directions", y=w272) -> (x = y?=w270:bool)
            n149 = Not(x=w270) -> (.not. x?=w271:bool)
            n150 = property on="Rev/Fwd" class="Clust (strict)"("Visible"=w270) -> ()  [unwired: 2 in, 2 out]
            n151 = property on="On/Off" class="Bool (strict)"("Visible"=w271, "Caption.Text"=w269) -> ()  [unwired: 2 in, 2 out]
          }
          frame "Compressor", "Digital Out" {
            w277 = FALSE ("Visible")
            # "Get direction and finish"
            n152 = property on="Motor" class="Clust (strict)"("Visible"=w277) -> ()  [unwired: 2 in, 2 out]
            n153 = property on="Test Slider" class="Slide (strict)"("Visible"=w277) -> ()  [unwired: 2 in, 2 out]
            n154 = property on="Test Ring" class="Ring (strict)"("Visible"=w277) -> ()  [unwired: 2 in, 2 out]
            n155 = property on="On/Off" class="Bool (strict)"("Visible"=TRUE, "Caption.Text"=w278) -> ()  [unwired: 2 in, 2 out]
            n156 = property on="Rev/Fwd" class="Clust (strict)"("Visible"=FALSE) -> ()  [unwired: 2 in, 2 out]
          }
          frame "Camera" {
            n157 = call <vilib>:"Get Last Path Segment.vi"("String in"=w285) -> ("String out"=w286:string)  [unwired: 10 in]
            n158 = property on="On/Off" class="Bool (strict)"("Visible"=FALSE) -> ()  [unwired: 2 in, 2 out]
            n159 = property on="Motor" class="Clust (strict)"("Visible"=FALSE) -> ()  [unwired: 2 in, 2 out]
            n160 = property on="Rev/Fwd" class="Clust (strict)"("Visible"=FALSE) -> ()  [unwired: 2 in, 2 out]
            n161 = case shown="\"White Balance  **\"" w286 {
              tunnel: w285 -> [w292 w301 w310 w319 w328 _ w334]
              tunnel: w284 -> [w290 w298 w307 w316 w325 _ _]
              frame "Size  **" {
                n162 = Index Array(array=w290) -> (element=w289:cluster{string[]})  [unwired: 1 in]
                n163 = call <vilib>:"NT Read String.vi"("Name"=w292) -> ("String"=w291:string)  [unwired: 9 in, 1 out]
                n164 = Unbundle(w289) -> (w287:string[])
                n165 = Match First String(2:w287, 3:w291) -> (0:w288:i32)  [unwired: 1 out]
                n166 = property on="Test Ring" class="Ring (strict)"("Value"=w288, "Strings []"=w287) -> ()  [unwired: 2 in, 2 out]
                n167 = property on="Test Ring" class="Ring (strict)"("Visible"=TRUE) -> ()  [unwired: 2 in, 2 out]
                n168 = property on="Test Slider" class="Slide (strict)"("Visible"=FALSE) -> ()  [unwired: 2 in, 2 out]
              }
              frame "White Balance  **" {
                n169 = Index Array(array=w298, index=1) -> (element=w299:cluster{string[]})
                n170 = call <vilib>:"NT Read String.vi"("Name"=w301) -> ("String"=w300:string)  [unwired: 9 in, 1 out]
                n171 = Unbundle(w299) -> (w296:string[])
                n172 = Match First String(2:w296, 3:w300) -> (0:w295:i32)  [unwired: 1 out]
                n173 = property on="Test Ring" class="Ring (strict)"("Value"=w295, "Strings []"=w296) -> ()  [unwired: 2 in, 2 out]
                n174 = property on="Test Ring" class="Ring (strict)"("Visible"=TRUE) -> ()  [unwired: 2 in, 2 out]
                n175 = property on="Test Slider" class="Slide (strict)"("Visible"=FALSE) -> ()  [unwired: 2 in, 2 out]
              }
              frame "Exposure  **" {
                n176 = Index Array(array=w307, index=2) -> (element=w308:cluster{string[]})
                n177 = call <vilib>:"NT Read String.vi"("Name"=w310) -> ("String"=w309:string)  [unwired: 9 in, 1 out]
                n178 = Unbundle(w308) -> (w304:string[])
                n179 = Match First String(2:w304, 3:w309) -> (0:w305:i32)  [unwired: 1 out]
                n180 = property on="Test Ring" class="Ring (strict)"("Value"=w305, "Strings []"=w304) -> ()  [unwired: 2 in, 2 out]
                n181 = property on="Test Ring" class="Ring (strict)"("Visible"=TRUE) -> ()  [unwired: 2 in, 2 out]
                n182 = property on="Test Slider" class="Slide (strict)"("Visible"=FALSE) -> ()  [unwired: 2 in, 2 out]
              }
              frame "Exposure Priority  **" {
                n183 = Index Array(array=w316, index=3) -> (element=w317:cluster{string[]})
                n184 = call <vilib>:"NT Read String.vi"("Name"=w319) -> ("String"=w318:string)  [unwired: 9 in, 1 out]
                n185 = Unbundle(w317) -> (w313:string[])
                n186 = Match First String(2:w313, 3:w318) -> (0:w314:i32)  [unwired: 1 out]
                n187 = property on="Test Ring" class="Ring (strict)"("Value"=w314, "Strings []"=w313) -> ()  [unwired: 2 in, 2 out]
                n188 = property on="Test Ring" class="Ring (strict)"("Visible"=TRUE) -> ()  [unwired: 2 in, 2 out]
                n189 = property on="Test Slider" class="Slide (strict)"("Visible"=FALSE) -> ()  [unwired: 2 in, 2 out]
              }
              frame "Color Enable  **" {
                n190 = Index Array(array=w325, index=4) -> (element=w326:cluster{string[]})
                n191 = call <vilib>:"NT Read String.vi"("Name"=w328) -> ("String"=w327:string)  [unwired: 9 in, 1 out]
                n192 = Unbundle(w326) -> (w322:string[])
                n193 = Match First String(2:w322, 3:w327) -> (0:w323:i32)  [unwired: 1 out]
                n194 = property on="Test Ring" class="Ring (strict)"("Value"=w323, "Strings []"=w322) -> ()  [unwired: 2 in, 2 out]
                n195 = property on="Test Ring" class="Ring (strict)"("Visible"=TRUE) -> ()  [unwired: 2 in, 2 out]
                n196 = property on="Test Slider" class="Slide (strict)"("Visible"=FALSE) -> ()  [unwired: 2 in, 2 out]
              }
              frame Default {
                n197 = property on="Test Ring" class="Ring (strict)"("Visible"=FALSE) -> ()  [unwired: 2 in, 2 out]
                n198 = property on="Test Slider" class="Slide (strict)"("Visible"=FALSE) -> ()  [unwired: 2 in, 2 out]
              }
              frame "Brightness  **", "Color Level  **", "Compression  **", "FPS  **", "Sharpness  **" {
                n199 = call <vilib>:"NT Read Number.vi"("Name"=w334) -> ("Numeric"=w333:dbl)  [unwired: 9 in, 1 out]
                n200 = local write "Test Slider"(w333) -> ()
                n201 = property on="Test Slider" class="Slide (strict)"("Visible"=TRUE, "Scale.Maximum"=100.0 ("Scale.Range:Maximum")) -> ()  [unwired: 2 in, 2 out]
                n202 = property on="Test Ring" class="Ring (strict)"("Visible"=FALSE) -> ()  [unwired: 2 in, 2 out]
              }
            }
          }
        }
        n203 = property on="Progress" class="Clust (strict)"("Visible"=FALSE) -> ()  [unwired: 2 in, 2 out]
      }
      event "Test Name": Mouse Enter {
        # "Populate the ring with the list of tests"
        n204 = event-data() -> ()  [unwired: 1 in, 1 out]
        n205 = call <vilib>:"NT Read String Array.vi"("Name"="/TestMode/TestList") -> ("String Array"=w343:string[])  [unwired: 9 in, 1 out]
        n206 = Build Array (concatenate)("Select the test to run...", w343) -> (w342:string[])
        n207 = property on="Test Name" class="Ring (strict)"("Strings []"=w342) -> ()  [unwired: 2 in, 2 out]
      }
      event "Test Name": Value Change {
        w346 = FALSE ("Visible")
        # "Tell the robot the test name to run"
        n208 = event-data() -> ("NewVal"=w350:u16)  [unwired: 1 in]
        n209 = property on="Test Name" class="Ring (strict)"() -> ("Strings []"=w351:string[])  [unwired: 2 in, 2 out]
        n210 = local write "Progress"(T7 {"Test Progress"=0, "Test Progress Text"=""} ("Progress")) -> ()
        n211 = Index Array(array=w351, index=w350) -> (element=w349:string)
        n212 = call <vilib>:"NT Write String.vi"("String"=w349, "Name"="/TestMode/TestName") -> ()  [unwired: 9 in, 1 out]
        n213 = property on="Progress" class="Clust (strict)"("Visible"=TRUE) -> ()  [unwired: 2 in, 2 out]
        n214 = property on="Motor" class="Clust (strict)"("Visible"=w346) -> ()  [unwired: 2 in, 2 out]
        n215 = property on="Test Slider" class="Slide (strict)"("Visible"=w346) -> ()  [unwired: 2 in, 2 out]
        n216 = property on="On/Off" class="Bool (strict)"("Visible"=w346) -> ()  [unwired: 2 in, 2 out]
        n217 = property on="Rev/Fwd" class="Clust (strict)"("Visible"=w346) -> ()  [unwired: 2 in, 2 out]
        n218 = property on="Test Ring" class="Ring (strict)"("Visible"=w346) -> ()  [unwired: 2 in, 2 out]
      }
      event "Select Auto": Mouse Enter {
        # "Populate the combo box with the list of autonomous options"
        n219 = event-data() -> ()  [unwired: 1 in, 1 out]
        n220 = call <vilib>:"NT Read String Array.vi"("Name"="Auto List") -> ("String Array"=w353:string[])  [unwired: 9 in, 1 out]
        n221 = property on="Select Auto" class="CmbBox"("Strings[]"=w353) -> ()  [unwired: 2 in, 2 out]
      }
      event "Select Auto": Value Change {
        # "User modified the Auto Selection. Write to NT variable so robot knows."
        n222 = event-data() -> ("NewVal"=w357:string)  [unwired: 1 in]
        n223 = call <vilib>:"NT Write String.vi"("String"=w357, "Name"="Auto Selector") -> ()  [unwired: 9 in, 1 out]
      }
      event "Command Selection": Value Change {
        # "Get the params and show in table"
        n224 = event-data() -> ("NewVal"=w364:i32)  [unwired: 1 in]
        n225 = property on="Command Selection" class="MCListbox (strict)"() -> ("ItemNames"=w362:string[][])  [unwired: 2 in, 2 out]
        n226 = call <vilib>:"WPI_DashboardUpdate Command Params.vi"("NewVal"=w364, "Commands"=w362, "Param Tbl"=w363) -> ()  [unwired: 8 in, 1 out]
      }
      event "Execute Command": Value Change {
        # "Started one, Unique ID holds\nresponse"
        n227 = event-data() -> ()  [unwired: 1 in, 1 out]
        n228 = property on="Command Selection" class="MCListbox (strict)"() -> ("ItemNames"=w376:string[][])  [unwired: 2 in, 2 out]
        n229 = Index Array(array=w376, index (row)="Command Selection", index (col)=0) -> (element=w374:string)
        n230 = call <vilib>:"Invoke Commands.vi"("Command Params"="Command Params", "Function Name"=w374) -> ("Params"=w370:u8, "Started"=w369:bool)  [unwired: 7 in, 1 out]
        n231 = Array Subset(array="Command Params", length (row)=w370) -> (w371:string[][])  [unwired: 3 in]
        n232 = Select(t="Executing" ("Cmd Status"), s=w369, f="" ("Cmd Status")) -> (s? t:f=→"Cmd Status":string)
      }
      event "Command Selection": Double Click {
        n233 = event-data() -> ("Row"=w386:i32)  [unwired: 1 in]
        n234 = property on="Command Selection" class="MCListbox (strict)"() -> ("ItemNames"=w389:string[][])  [unwired: 2 in, 2 out]
        n235 = local read "Command Params"() -> (w384:string[][])
        n236 = Index Array(array=w389, index (row)=w386, index (col)=0) -> (element=w387:string)
        n237 = call <vilib>:"Invoke Commands.vi"("Command Params"=w384, "Function Name"=w387) -> ("Params"=w383:u8, "Started"=w378:bool)  [unwired: 7 in, 1 out]
        n238 = Array Subset(array=w384, length (row)=w383) -> (w382:string[][])  [unwired: 3 in]
        n239 = Select(t="Executing" ("Cmd Status"), s=w378, f="" ("Cmd Status")) -> (s? t:f=w379:string)
        n240 = local write "Cmd Status"(w379) -> ()
      }
      event "CheckList": Double Click {
        # "Shift clears all"
        # "Update symbols on the listbox"
        n241 = event-data() -> ("PlatMods.Shift"=w392:bool, "Row"=w394:i32)  [unwired: 1 in]
        n242 = case shown="True" w392 {
          tunnel: w394 -> [w398 _]
          tunnel: 1 -> [w397 _]
          frame False {
            n243 = property on="CheckList" class="LstBox (strict)"() -> ("Item Symbols"=w396:i32[])  [unwired: 2 in, 2 out]
            n244 = Replace Array Subset(array=w396, new element=w397, index=w398) -> (w395:i32[])
            n245 = property on="CheckList" class="LstBox (strict)"("Item Symbols"=w395) -> ()  [unwired: 2 in, 2 out]
          }
          frame True {
            w399 = 0 ("Top Row")
            n246 = property on="CheckList" class="LstBox (strict)"() -> ("Number of Rows"=w401:u32)  [unwired: 2 in, 2 out]
            n247 = Initialize Array(0, w401) -> (w400:i32[])
            n248 = property on="CheckList" class="LstBox (strict)"("Top Row"=w399, "Value"=w399, "Item Symbols"=w400) -> ()  [unwired: 2 in, 2 out]
          }
        }
      }
      event "CheckList": Key Down {
        # "Update symbols on the listbox\nLeft and right keys check and uncheck"
        n249 = event-data() -> ("VKey"=w406:T21)  [unwired: 1 in]
        n250 = case shown="\"Left\", \"Right\"" w406 {
          selector: w406 -> [w411 _]
          tunnel: eventvkey."Left" ("VKey") -> [w409 _]
          frame "Left", "Right" {
            n251 = Equal?(x=w409, y=w411) -> (x = y?=w410:bool)
            n252 = Select(t=0, s=w410, f=1) -> (s? t:f=w412:i32)
            n253 = property on="CheckList" class="LstBox (strict)"() -> ("Item Symbols"=w415:i32[])  [unwired: 2 in, 2 out]
            n254 = Replace Array Subset(array=w415, new element=w412, index="CheckList") -> (w414:i32[])
            n255 = property on="CheckList" class="LstBox (strict)"("Item Symbols"=w414) -> ()  [unwired: 2 in, 2 out]
          }
          frame Default {
          }
        }
      }
      event "DB Camera Config": Value Change {
        # "Show or hide the cluster of controls, store in ini file"
        n256 = event-data() -> ("NewVal"=w420:bool)  [unwired: 1 in]
        n257 = case shown="False" w420 {
          tunnel: w419 -> [w429 _]
          tunnel: [w422 w440] -> w418
          tunnel: w417 -> [w421 w440]
          frame False {
            w436 = "Camera"
            w439 = FALSE ("Visible")
            n258 = local read "Camera Settings"() -> (w428:T2)
            n259 = Index Array(array=w429) -> (element=w432:cluster{string[]})  [unwired: 1 in]
            n260 = Unbundle(w428) -> ("Frame Rate"=w427:i32, "Compression"=w426:i32, "Size"=w430:u16)
            n261 = Unbundle(w432) -> (w431:string[])
            n262 = Index Array(array=w431, index=w430) -> (element=w425:string)
            n263 = call-poly <vilib>:"Write Key.vi"("section"=w436, "value"=w425, "key"="Size", "refnum"=w421) -> ("refnum out"=w438:T19)  [unwired: 2 in, 5 out]
            n264 = call-poly <vilib>:"Write Key.vi"("section"=w436, "value"=w427, "key"="FrameRate", "refnum"=w438) -> ("refnum out"=w437:T19)  [unwired: 1 in, 6 out]
            n265 = property on="Camera Settings" class="Clust (strict)"("Visible"=w439) -> ()  [unwired: 2 in, 2 out]
            n266 = local write "DB Camera Config"(w439) -> ()
            n267 = call-poly <vilib>:"Write Key.vi"("section"=w436, "value"=w426, "key"="Compression", "refnum"=w437) -> ("refnum out"=w423:T19)  [unwired: 1 in, 6 out]
            n268 = call <vilib>:"Close Config Data.vi"("refnum"=w423) -> ("file path"=w424:path)  [unwired: 2 in, 8 out]
            n269 = call <vilib>:"Open Config Data.vi"("configuration file path"=w424) -> ("refnum"=w422:T19)  [unwired: 8 in, 2 out]
          }
          frame True {
            n270 = property on="Camera Settings" class="Clust (strict)"("Visible"=TRUE) -> ()  [unwired: 2 in, 2 out]
          }
        }
      }
      event "Camera Settings": Value Change {
        # "Update summary string when any elements of DB camera change"
        n271 = event-data() -> ("NewVal"=w454:T2)  [unwired: 1 in]
        n272 = Index Array(array=w450) -> (element=w449:cluster{string[]})  [unwired: 1 in]
        n273 = Unbundle(w454) -> ("Frame Rate"=w445:i32, "Compression"=w444:i32, "Size"=w447:u16)
        n274 = Unbundle(w449) -> (w448:string[])
        n275 = Index Array(array=w448, index=w447) -> (element=w446:string)
        n276 = Format Into String(format string="%s   %dfps   %d%%", w446, w445, w444) -> (resulting string=w451:string)  [unwired: 2 in, 1 out]
        n277 = Build Array(w451) -> (w452:string[])
        n278 = property on="DB Camera Config" class="Bool (strict)"("Strings [4]"=w452) -> ()  [unwired: 2 in, 2 out]
      }
      event "Motor.Enable": Value Change {
        # "When the test mode otor enable helper is set, update that\ntree row item's value"
        n279 = event-data() -> ("NewVal"=w461:bool)  [unwired: 1 in]
        n280 = Unbundle("Motor") -> ("Value"=w460:dbl)  [unwired: 1 out]
        n281 = Select(t=w460, s=w461, f=0.0) -> (s? t:f=w458:dbl)
        n282 = call <vilib>:"NT Write Number.vi"("Numeric"=w458, "Name"=w457) -> ()  [unwired: 9 in, 1 out]
      }
      event "Test Slider": Value Change {
        # "When the test mode slider helper is set, update that\ntree row item's value"
        n283 = event-data() -> ("NewVal"=w465:dbl)  [unwired: 1 in]
        n284 = call <vilib>:"NT Write Number.vi"("Numeric"=w465, "Name"=w466) -> ()  [unwired: 9 in, 1 out]
      }
      event "On/Off": Value Change {
        # "When the test mode on/off helper value is set, update that\ntree row item's value"
        n285 = event-data() -> ("NewVal"=w471:bool)  [unwired: 1 in]
        n286 = Boolean To (0,1)(Boolean=w471) -> (0, 1=w470:i16)
        n287 = call <vilib>:"NT Write Number.vi"("Numeric"=w470, "Name"=w469) -> ()  [unwired: 9 in, 1 out]
      }
      event "Rev/Fwd": Value Change {
        # "When the test mode helper value for relays is set, update that\ntree row item's value"
        n288 = event-data() -> ("NewVal.Forward"=w480:bool, "NewVal.Reverse"=w479:bool)  [unwired: 1 in]
        n289 = Boolean To (0,1)(Boolean=w480) -> (0, 1=w476:i16)
        n290 = Boolean To (0,1)(Boolean=w479) -> (0, 1=w478:i16)
        n291 = Negate(x=w478) -> (-x=w477:i16)
        n292 = Add(x=w476, y=w477) -> (x+y=w475:i16)
        n293 = call <vilib>:"NT Write Number.vi"("Numeric"=w475, "Name"=w474) -> ()  [unwired: 9 in, 1 out]
      }
      event "Test Ring": Value Change {
        # "When a test mode helper value is selected from the ring,\nset the tree item's variable to the string value"
        n294 = event-data() -> ("NewVal"=w485:u16)  [unwired: 1 in]
        n295 = property on="Test Ring" class="Ring (strict)"() -> ("Strings []"=w486:string[])  [unwired: 2 in, 2 out]
        n296 = Index Array(array=w486, index=w485) -> (element=w484:string)
        n297 = call <vilib>:"NT Write String.vi"("String"=w484, "Name"=w483) -> ()  [unwired: 9 in, 1 out]
      }
      event "Rec Mode": Value Change {
        # "Update globals for recording mode and path to read log from.\nClear when logging and let NetworkTables set path for vision to\nuse."
        n298 = event-data() -> ("NewVal"=w498:enum32{"Stop", "Record", "Playback"})  [unwired: 1 in]
        n299 = global write "WPI_DashboardLogging Global.vi" "Logging Filename"(path "") -> ()
        n300 = global write "WPI_DashboardLogging Global.vi" "Recording"(w498) -> ()
        n301 = case shown="\"Playback\"" w498 {
          tunnel: w497 -> [_ w500 w509]
          tunnel: [_ _ w508] -> w494
          tunnel: [_ _ w507] -> _
          tunnel: w492 -> [_ _ w505]
          tunnel: cluster{i32, i32} {-250, 170} -> [_ _ w504]
          tunnel: [_ _ T22 {"Image Size"=TRUE, "Image Type"=TRUE, "Pixel Value"=TRUE, "ROI Information"=TRUE, "Zoom Factor"=FALSE} ("Image Information Shown:All Elements")] -> w490
          tunnel: [_ _ TRUE ("Zoom Factor")] -> w489
          tunnel: w488 -> [_ _ w501]
          frame Default {
          }
          frame "Stop", "Record" {
            # "Place Window too"
            n302 = invoke class="VI" method="FP.Close"(reference=w500) -> (reference out=w499:refnum<vi>)  [unwired: 2 in, 2 out]
            n303 = invoke class="VI" method="Abort VI"(reference=w499) -> ()  [unwired: 2 in, 3 out]
          }
          frame "Playback" {
            n304 = call "Open Playback Panel.vi"("Offset"=w504, "DB VI Ref"=w505, "Playback in"=w509) -> ("Playback out"=w506:refnum<vi>)  [unwired: 8 in]
            n305 = register-events(w506, w501) -> (reference out=w508:refnum<event-registration>, error out=w507:errorcluster)  [unwired: 2 in]
          }
        }
        n306 = property on="Camera Image" class="ImageControl"("Image Information Shown"=w490, "Image Information Visible"=w489) -> ()  [unwired: 2 in, 2 out]
        n307 = call <vilib>:"WPI_DashboardNT Log FieldName Cache.vi"("Operation"=enum16{"Lookup/Add", "Index", "Clear"}."Clear") -> ()  [unwired: 8 in, 3 out]
      }
      event Panel Close {
        w511 = enum32{"Stop", "Record", "Playback"}."Stop" ("Rec Mode")
        # "Playback window has been closed, abort"
        n308 = event-data() -> ()  [unwired: 1 in, 4 out]
        n309 = local write "Rec Mode"(w511) -> ()
        n310 = global write "WPI_DashboardLogging Global.vi" "Recording"(w511) -> ()
      }
      event Panel Close {
        # "Abort playback window and ourself"
        n311 = event-data() -> ()  [unwired: 1 in, 4 out]
        n312 = invoke class="VI" method="FP.Close"(reference=w517) -> (reference out=w516:refnum<vi>)  [unwired: 2 in, 2 out]
        n313 = invoke class="VI" method="Abort VI"(reference=w516) -> (error out=w515:errorcluster)  [unwired: 2 in, 2 out]
        n314 = invoke class="VI" method="Abort VI"(error in=w515) -> ()  [unwired: 2 in, 3 out]
      }
      event User Event {
        n315 = event-data() -> ("IDs"=w525:cluster{"RPC field ID":u16, "Unique ID":u16}, "String"=w524:string)  [unwired: 1 in]
        n316 = Bundle("IDs"=w525, "String"=w524) -> (w523:T9)  [unwired: 1 in]
        n317 = call <vilib>:"Retrieve RPC Response.vi"("RPC Response"=w523) -> ("Output"=w520:string[][])  [unwired: 10 in]
        n318 = Build Array (concatenate)(w518, w520) -> (w519:string[][])
        n319 = local write "Command Params"(w519) -> ()
        n320 = local write "Cmd Status"("" ("Cmd Status")) -> ()
      }
      event "Vision": Value Change {
        # "Enable/Disable Compression slider.\nHW USB is hard-coded into the camera"
        n321 = event-data() -> ("NewVal"=w532:u16)  [unwired: 1 in]
        n322 = Equal?(x=w532, y=u32 2 ("milliseconds to wait")) -> (x = y?=w530:bool)
        n323 = Select(t=T23."Disabled and Grayed Out" ("Disabled"), s=w530, f=T23."Enabled" ("Disabled")) -> (s? t:f=w527:T23)
        n324 = property on="Compression" class="Slide (strict)"("DisabledEnum"=w527) -> ()  [unwired: 2 in, 2 out]
      }
      event "Tree": Double Click {
        n325 = event-data() -> ("PlatMods"=w537:T26, "Tag"=w536:string)  [unwired: 1 in]
        n326 = Unbundle(w537) -> ("Shift"=w535:bool)  [unwired: 4 out]
        n327 = Not(x=w535) -> (.not. x?=w534:bool)
        n328 = call <vilib>:"NT Update Persistence.vi"("Persistence"=w534, "Name"=w536) -> ()  [unwired: 9 in, 1 out]
      }
    }
  }
  n329 = while {
    tunnel: w51 -> [w541]
    i -> [w544]
    stop <- FALSE stop-if-true
    n330 = Wait (ms)(milliseconds to wait=u32 100) -> ()  [unwired: 1 out]
    n331 = case shown="\"Playback\"" "Rec Mode" {
      tunnel: w544 -> [_ _ w559]
      tunnel: [u32 2829099 ("Base Color") u32 11141120 ("Target Color") w548] -> w540
      frame "Stop", Default {
        # "Reset the color, extra updates don't cost much"
      }
      frame "Record" {
      }
      frame "Playback" {
        # "Playback"
        n332 = Quotient & Remainder(x=w559, y=u32 50 ("milliseconds to wait")) -> (x-y*floor(x/y)=w555:u32)  [unwired: 1 out]
        n333 = Divide(x=w555, y=u32 50 ("milliseconds to wait")) -> (x/y=w552:dbl)
        n334 = Multiply(x=6.283185307179586, y=w552) -> (x*y=w557:dbl)
        n335 = Sine(x=w557) -> (sin(x)=w556:dbl)
        n336 = Absolute Value(x=w556) -> (abs(x)=w549:dbl)
        n337 = call "Interpolate RGB Color.vi"("Proportion"=w549, "Target Color"=u32 30976, "Base Color"=u32 2829099) -> ("Result Color"=w548:u32)  [unwired: 8 in]
      }
    }
    n338 = property class="Pane"(reference=w541, "PaneColor"=w540) -> ()  [unwired: 1 in, 2 out]
  }
  n339 = local write "Dashboard Tab"(T1."Drive" ("Dashboard Tab")) -> ()
  n340 = property on="On/Off" class="Bool (strict)"("Visible"=w22) -> ()  [unwired: 2 in, 2 out]
  n341 = property on="Motor" class="Clust (strict)"("Visible"=w22) -> ()  [unwired: 2 in, 2 out]
  n342 = property on="Progress" class="Clust (strict)"("Visible"=w22) -> ()  [unwired: 2 in, 2 out]
  n343 = property on="Test Ring" class="Ring (strict)"("Visible"=w22) -> ()  [unwired: 2 in, 2 out]
  n344 = property on="Rev/Fwd" class="Clust (strict)"("Visible"=w22) -> ()  [unwired: 2 in, 2 out]
  n345 = property on="Camera Settings" class="Clust (strict)"("Visible"=w22) -> ()  [unwired: 2 in, 2 out]
  n346 = while {
    tunnel: u16 1741 ("timeout ms (25000)") -> [w561]
    stop <- FALSE stop-if-true
    n347 = TCP Create Listener(10:w561) -> (0:w560:errorcluster, 3:w562:refnum<k5>)  [unwired: 4 in, 1 out]
    n348 = case shown="No Error" w560 {
      selector: w560 -> [w564 _]
      tunnel: w562 -> [w565 _]
      frame No Error {
        n349 = while {
          tunnel: w565 -> [w568]
          tunnel: w564 -> [w567]
          stop <- FALSE stop-if-true
          n350 = TCP Wait On Listener(8:w567, 11:w568) -> (0:w569:errorcluster, 4:w570:refnum<k5>)  [unwired: 2 in, 3 out]
          n351 = local write "TCP"(w570) -> ()
          n352 = case shown="No Error" w569 {
            frame No Error {
            }
            frame Error {
              n353 = Wait (ms)(milliseconds to wait=u32 1000) -> ()  [unwired: 1 out]
            }
          }
        }
      }
      frame Error {
        n354 = Wait (ms)(milliseconds to wait=u32 1000) -> ()  [unwired: 1 out]
      }
    }
  }
  n355 = local write "DB Camera Config"(w22) -> ()
  n356 = local write "Command Params"(string[][] [] ("Command Params")) -> ()
  n357 = global write "WPI_DashboardLogging Global.vi" "Recording"(w45) -> ()
  n358 = local write "Command Selection"(u16 0 ("milliseconds to wait")) -> ()
  n359 = local write "Rec Mode"(w45) -> ()
